vi "PI Terminal.vi"() -> ()   [LabVIEW 2014]
doc: "HELP for Terminal.vi\n\nThe terminal VI is a stand-alone application. It first asks the user to specify the full configuration (number of controlled systems, RS-232, GPIB, TCP-IP or DLL communication, communications parameters), then it establishes a connection with a selected system. This will work for all PI devices which support the PI General Command Set, or at least follow the same syntax rules and support the *IDN? and ERR? commands.\n\nAfter starting the VI, the interface parameters of the systems with which to communicate must be selected. For this reason, \"PITerminal.vi\" calls \"PI Ask for Communication Parameters.vi\". Select here the number of connected PI systems that you want to communicate with. For each system, select the appropriate interface parameters. \n\nC-413: Interface = RS232, DLL, or TCP/IP. TCP/IP support available depending on controller version! If unsure whether your controller supports TCP/IP communication, please refer to the controller user manual), RS232: Input and output HW handshake must be TRUE. DLL: DLL for Device = PI_GCS2_DLL, DLL Interface = USB, Parameter = Serial no. of system to connect to. Syntax: GCS 2.0; Term char = LF.\n\nC-702: Interface = RS232 or TCP/IP, RS232: Input and output HW handshake must be TRUE. Syntax: GCS 1.0; Term char = LF.\n\nC-843: Interface = DLL, DLL for Device = C-843, DLL Interface = Board, Parameter = Board number (1 for first C-843 board). Syntax: GCS 1.0; Term char = LF.\n\nC-843.PM: Interface = DLL, DLL for Device = C-843.PM, DLL Interface = Board, Parameter = Board number (1 for first C-843 board). Syntax: GCS 1.0; Term char = LF.\n\nC-844: Interface = DLL, DLL for Device = C-844, DLL Interface = RS232 or GPIB, Parameter = empty string, RS232 baud rate = 9600. Syntax: GCS 1.0; Term char = LF.\n\nC-865: Interface = DLL, DLL for Device = C-865, DLL Interface = RS232, Parameter = empty string, RS232 baud rate = set as appropriate. Syntax: GCS 1.0; Term char = LF.\n\nC-866: Interface = DLL, DLL for Device = C-866, DLL Interface = RS232 or USB, RS232: Parameter = empty string, RS232 baud rate = set as appropriate, USB: Parameter = Serial no. of system to connect to, Syntax: GCS 1.0; Term char = LF.\n\nC-867: Single Device: Interface = RS232, TCP/IP or DLL, RS232: Input and output HW handshake must be FALSE. DLL (USB): DLL for Device = C-867, DLL Interface = USB, Parameter = Serial no. of system to connect to. DaisyChain: Interface = DLL, DLL for Device = C-867, DLL Interface = RS232_DC, Parameter = Number of device in chain, Register DC: FALSE. Syntax: GCS 2.0; Term char = LF.\n\nC-877: Interface = RS232 or DLL, RS232: Input and output HW handshake must be FALSE. DLL (USB): DLL for Device = PI_GCS2_DLL, DLL Interface = USB, Parameter = Serial no. of system to connect to. Syntax: GCS 2.0; Term char = LF.\n\nC-880, C-848: Interface = RS232 or GPIB, RS232: Input and output HW handshake must be TRUE. Syntax: GCS 1.0; Term char = LF.\n\nC-880K005: Interface = RS232, Input and output HW handshake must be FALSE. Syntax: GCS 1.0; Term char = LF.\n\nC-884: Interface = RS232, TCP/IP or DLL, RS232: Input and output HW handshake must be FALSE. DLL (USB): DLL for Device = PI_GCS2_DLL, DLL Interface = USB, Parameter = Serial no. of system to connect to. Syntax: GCS 2.0; Term char = LF.\n\nC-885: Interface = TCP/IP or DLL. DLL (USB): DLL for Device = PI_GCS2_DLL, DLL Interface = USB, Parameter = Serial no. of system to connect to. Syntax: GCS 2.0; Term char = LF.DaisyChain: Interface = DLL, DLL for Device = PI_GCS2_DLL, DLL Interface = TCPIP_DC or USB_DC, Parameter = Number of device in chain, Register DC: FALSE. Syntax: GCS 2.0; Term char = LF.\n\nC-886: Interface = TCP/IP or DLL. DLL (USB): DLL for Device = PI_GCS2_DLL, DLL Interface = USB, Parameter = Serial no. of system to connect to. Syntax: GCS 2.0; Term char = LF.\n\nC-887, F-206, M-8X0: For GCS syntax version = GCS 1.0 (older firmware or compatibility mode, can be set with CSV.vi), Interface = RS232, GPIB (not available for C-887 controller) or TCP/IP., The error status will not be cleared by this VI. The first ERR? query will report a hidden error with error code 1, which will be cleared during system initialization (INI). RS232: Input and output handshake settings must be FALSE. Syntax: GCS 1.0; Term char = LF.\nFor GCS syntax version = GCS 2.0 (C-887 Controller), Interface = RS232 or TCP/IP. RS232: Input and output handshake settings must be FALSE. Syntax: GCS 2.0; Term char = LF.\n\nC-891: Interface = RS232, TCP/IP or DLL. TCP/IP support available depending on controller version! If unsure whether your controller supports TCP/IP communication, please refer to your user manual. RS232: Input and output HW handshake must be FALSE. DLL (USB): DLL for Device = PI_GCS2_DLL, DLL Interface = USB, Parameter = Serial no. of system to connect to. Syntax: GCS 2.0; Term char = LF.\n\nE-516: Interface = RS232 or GPIB, RS232: Input and output HW handshake must be TRUE. Syntax: GCS 1.0; Term char = LF.\n\nE-517: Interface = RS232, GPIB, TCP/IP or DLL, RS232: Input and output HW handshake must be TRUE, DLL (USB): DLL for Device = E-517, DLL Interface = USB, Parameter = Serial no. of system to connect to. Syntax: GCS 2.0; Term char = LF.\n\nE-518: Interface = RS232, TCP/IP or DLL, RS232: Input and output HW handshake must be TRUE, DLL (USB): DLL for Device = PI_GCS2_DLL, DLL Interface = USB, Parameter = Serial no. of system to connect to. Syntax: GCS 2.0; Term char = LF.\n\nE-709: Interface = RS232 or DLL, RS232: Input and output HW handshake must be TRUE. DLL (USB): DLL for Device = E-709, DLL Interface = USB, Parameter = Serial no. of system to connect to. Syntax: GCS 2.0; Term char = LF.\n\nE-710: Interface = DLL, DLL for Device = E-710, DLL Interface = RS232 or GPIB, Parameter = empty string. Syntax: GCS 1.0; Term char = LF.\n\nE-712: Interface = RS232, TCP/IP or DLL, RS232: Input and output HW handshake must be TRUE. DLL: DLL for Device = E-712, DLL Interface = USB, Parameter = Serial no. of system to connect to. Syntax: GCS 2.0; Term char = LF.\n\nE-725: Interface = RS232, TCP/IP or DLL, RS232: Input and output HW handshake must be TRUE. DLL: DLL for Device = E-725, DLL Interface = USB, Parameter = Serial no. of system to connect to. Syntax: GCS 2.0; Term char = LF.\n\nE-727: Interface = RS232, TCP/IP or DLL, RS232: Input and output HW handshake must be TRUE. DLL: DLL for Device = PI_GCS2_DLL, DLL Interface = USB,Parameter = Serial no. of system to connect to. Syntax: GCS 2.0; Term char = LF.\n\nE-753: Interface = RS232 or TCP/IP, RS232: Input and output HW handshake must be TRUE. Syntax: GCS 2.0; Term char = LF.\n\nE-754: Interface = RS232, TCP/IP or DLL, RS232: Input and output HW handshake must be TRUE. DLL: DLL for Device = E-754, DLL Interface = USB, Parameter = Serial no. of system to connect to. Syntax: GCS 2.0; Term char = LF.\n\nE-755: Single Device: Interface = RS232, Input and output HW handshake must be TRUE. DaisyChain: Interface = DLL, DLL for Device = E-755, DLL Interface = RS232_DC, Parameter = Number of device in chain (first device: 1). Syntax: GCS 2.0; Term char = LF.\n\nE-761: Interface = DLL, DLL for Device = E-761, DLL Interface = Board, Parameter = Board number (1 for first E-761 board). Syntax: GCS 1.0; Term char = LF.\n\nE-816: Interface = RS232 or DLL, RS232: Input and output HW handshake must be TRUE. DLL (USB): DLL for Device = E-816, DLL Interface = USB, Parameter = Serial no. of system to connect to. Syntax: GCS 1.0; Term char = LF. \n\nE-861: Single Device: Interface = RS232 or DLL, RS232: Input and output HW handshake must be FALSE. DLL (USB): DLL for Device = E-861, DLL Interface = USB, Parameter = Serial no. of system to connect to. DaisyChain: Interface = DLL, DLL for Device = E-861, DLL Interface = RS232_DC, Parameter = Number of device in chain (first device: 1), Register DC: FALSE. Syntax: GCS 2.0; Term char = LF.\n\nE-870: Interface = DLL, DLL (USB): DLL for Device = PI_GCS2_DLL, DLL Interface = USB, Parameter = Serial no. of system to connect to.\nSyntax: GCS 2.0; Term char = LF.\n\nE-871: Single Device: Interface = RS232 or DLL, RS232: Input and output HW handshake must be FALSE. DLL (USB): DLL for Device = PI_GCS2_DLL, DLL Interface = USB, Parameter = Serial no. of system to connect to.\nDaisyChain: Interface = DLL, DLL for Device = PI_GCS2_DLL, DLL Interface = RS232_DC or USB_DC, Parameter = Number of device in chain, Register DC: FALSE. Syntax: GCS 2.0; Term char = LF.\n\nE-872: Interface = RS232, TCP/IP or DLL, RS232: Input and output HW handshake must be FALSE. DLL (USB): DLL for Device = PI_GCS2_DLL, DLL Interface = USB, Parameter = Serial no. of system to connect to. Syntax: GCS 2.0; Term char = LF.\n\nE-873: Interface = RS232, TCP/IP or DLL, RS232: Input and output HW handshake must be FALSE. DLL (USB): DLL for Device = PI_GCS2_DLL, DLL Interface = USB, Parameter = Serial no. of system to connect to. Syntax: GCS 2.0; Term char = LF.\n\nE-874: Interface = RS232, TCP/IP or DLL, RS232: Input and output HW handshake must be FALSE. DLL (USB): DLL for Device = PI_GCS2_DLL, DLL Interface = USB, Parameter = Serial no. of system to connect to. Syntax: GCS 2.0; Term char = LF.\n\nHydra: Interface = DLL, DLL (TCP/IP and RS-232): DLL for Device = PI_HydraPollux_GCS2_DLL, DLL Interface = RS232 or TCP/IP, Syntax: GCS 2.0; Term char = LF.\n\nMercury™: Interface = DLL, DLL for Device = Mercury™, DLL Interface = RS232 (even if using USB), Parameter = empty string, RS232 baud rate = same as set on controller hardware. Syntax: GCS 1.0; Term char = LF.\n\nGCS_Mercury: Single Device: Interface = RS232 or DLL, RS232: Input and output HW handshake must be FALSE. DLL (USB): DLL for Device = PI_GCS2_DLL, DLL Interface = USB, Parameter = Serial no. of system to connect to.\nDaisyChain: Interface = DLL, DLL for Device = PI_GCS2_DLL, DLL Interface = RS232_DC, Parameter = Number of device in chain, Register DC: FALSE. Syntax: GCS 2.0; Term char = LF.\n\nPollux: Interface = DLL, DLL (RS-232): DLL for Device = PI_HydraPollux_GCS2_DLL, DLL Interface = RS232, Baudrate must be 19200, Syntax: GCS 2.0; Term char = LF.\n\nIf the chosen timeout value is greater than 1000 ms, it will automatically be set to 1000 ms for a fluid program operation. \n\nIn the upper window (\"Send\") the user can enter commands which will be transmitted to the chosen device one line at a time when the ENTER key is pressed. \nAll controller responses are displayed in the Receive response window, which can be cleared by pressing the Clear Receive Window button or F2. \n\nThe view style of the Receive window can be changed to Show all characters or Hex View using the menu ring above the Receive window.\n\nExit or F10 will terminate the terminal application. \n\nTo send the last command again, just press the ENTER key again. The next line will then show the following entry: \"(Send: cmd)\" with cmd being the command from the line before, which was resent.\n\nWhen the terminal application has just been started, pressing ENTER without entering a command will send \"*IDN?\" to the chosen system. \n\nNew commands can only be inserted into the last line of the Send window. The user can scroll through the history of the Send window using the scroll bar or the cursor up/down keys, but cannot change the history or resend commands by pressing ENTER unless in the last line. Pressing ENTER will always resend the last command, no matter where the cursor is positioned. Selecting text and using copy and paste (Ctrl+C, Ctrl+V) works for single lines, if only the contents of one single line (the command text) is selected and copied, not the full line (including the LineFeed) or multiple lines.\n\nMany of PI's General Command Set compatible devices support single-byte commands. For example, the user can stop a fast scan of a C-880 or C-887by sending an ASCII 24 (decimal). To enter this command into the Send window simply type a \"#\" followed by the decimal value of the byte to be sent, e.g. enter \"#24\" and presses ENTER to stop a fast scan. An entry \"(Send: *)\" will be added to the original command with * being the corresponding ASCII character of the single byte sent. \n\nPressing F1 or the Help button will pop up a help window. To return to the terminal application, press Esc. If Send ERR? on Exit? is TRUE, an \"ERR?\" query is sent to the device when Exit is pressed to prevent the controller from keeping an error condition produced during the use of the terminal application."
uses:
  Low Level/Communication.llb/Termination character.ctl
  Low Level/Communication.llb/Available DLLs.ctl
  Low Level/Communication.llb/Global DaisyChain.vi
panel:
  out "Help string":string="\nHELP for PI Terminal.vi\nPress Esc to return to the terminal application.\n\nThis terminal application works for all PI devices which support the PI General Command Set or at least follow the syntax rules of this command structure and support the commands *IDN? and ERR?.\n\nIn the upper window (\"Send\") the user can enter commands which will be transmitted to the chosen device one line at a time when the ENTER key is pressed. All controller responses are displayed in the Receive response window, which can be cleared by pressing the Clear Receive Window button or F2. The view style of the Receive window can be changed to Show all characters or Hex View using the menu ring above the Receive window.\n\nExit or F10 will terminate the terminal application. \n\nTo send the last command again, just press the ENTER key again. The next line will then show the following entry: \"(Send: cmd)\" with cmd being the command from the line before, which was resent.\nWhen the terminal application has just been started, pressing ENTER without entering a command will send \"*IDN?\" to the chosen system.\n\nNew commands can only be inserted into the last line of the Send window. The user can scroll through the history of the Send window using the scroll bar or the cursor up/down keys, but cannot change the history or resend commands by pressing ENTER unless in the last line. Pressing ENTER will always resend the last command, no matter where the cursor is positioned. Selecting text and using copy and paste (Ctrl+C, Ctrl+V) works for single lines, if only the contents of one single line (the command text) is selected and copied, not the full line (including the LineFeed) or multiple lines.\n\nMany of PI's General Command Set compatible devices support single-byte commands. For example, the user can stop a fast scan of a C-880 or F-206 by sending an ASCII 24 (decimal). To enter this command into the Send window simply type a \"#\" followed by the decimal value of the byte to be sent, e.g. enter \"#24\" and presses ENTER to stop a fast scan. An entry \"(Send: *)\" will be added to the original command with * being the corresponding ASCII character of the single byte sent. \n\nIf Send ERR? on Exit? is TRUE, a \"ERR?\" query is sent to the device when Exit is pressed to prevent the controller from keeping an error condition produced during the use of the terminal application.\n\nC-413: \tInterface = RS232, DLL, or TCP/IP. TCP/IP support available depending on controller version! If unsure whether your controller supports TCP/IP communication, please refer to the controller user manual), RS232: Input and output HW handshake must be TRUE. DLL: DLL for Device = PI_GCS2_DLL, DLL Interface = USB, Parameter = Serial no. of system to connect to. Syntax: GCS 2.0; Term char = LF.\n\nC-414: \tInterface = RS232, DLL, or TCP/IP. RS232: Input and output HW handshake must be TRUE. DLL: DLL for Device = PI_GCS2_DLL, DLL Interface = USB, Parameter = Serial no. of system to connect to. Syntax: GCS 2.0; Term char = LF.\n\nC-702: \tInterface = RS232 or TCP/IP, RS232: Input and output HW handshake \tmust \tbe TRUE. Syntax: GCS 1.0; Term char = LF.\n\nC-843: \tInterface = DLL, DLL for Device = C-843, DLL Interface = Board, \tParameter = Board number (1 for first C-843 board). Syntax: GCS 1.0; \tTerm char = LF.\n\nC-843.PM: \tInterface = DLL, DLL for Device = C-843.PM, DLL Interface = Board, \tParameter = Board number (1 for first C-843 board). Syntax: GCS 1.0; \tTerm char = LF.\n\nC-865: \tInterface = DLL, DLL for Device = C-865, DLL Interface = RS232, \tParameter = empty string, RS232 baud rate = set as appropriate. Syntax: \tGCS 1.0; Term char = LF.\n\nC-866: \tInterface = DLL, DLL for Device = C-866, DLL Interface = RS232 or USB, \tRS232: Parameter = empty string, RS232 baud rate = set as appropriate, \tUSB: Parameter = Serial no. of system to connect to, \n\tSyntax: GCS 1.0; Term char = LF.\n\nC-867: \tSingle Device: Interface = RS232, TCP/IP or DLL, RS232: Input and output HW \thandshake must be FALSE. DLL (USB): DLL for Device = C-867, DLL \tInterface = USB, Parameter = Serial no. of system to connect to.\nDaisyChain: Interface = DLL, DLL for Device = C-867, DLL Interface = \tRS232_DC, Parameter = Number of device in chain, \tRegister DC: \tFALSE. Syntax: GCS 2.0; Term char = LF.\n\nC-880, C-848: \tInterface = RS232 or GPIB, RS232: Input and output HW handshake must \tbe TRUE. Syntax: GCS 1.0; Term char = LF.\n\nC-880K005: \tInterface = RS232, Input and output HW handshake must be FALSE. \tSyntax: GCS 1.0; Term char = LF.\n\nC-884: \tInterface = RS232, TCP/IP or DLL, RS232: Input and output HW handshake must be FALSE. DLL (USB): DLL for Device = PI_GCS2_DLL, DLL Interface = USB, Parameter = Serial no. of system to connect to. Syntax: GCS 2.0; Term char = LF.\n\nC-885: \tInterface = TCP/IP or DLL. DLL (USB): DLL for Device = PI_GCS2_DLL, DLL Interface = USB, Parameter = Serial no. of system to connect to. Syntax: GCS 2.0; Term char = LF.\nDaisyChain: Interface = DLL, DLL for Device = PI_GCS2_DLL, DLL Interface = \tTCPIP_DC or USB_DC, Parameter = Number of device in chain, \tRegister DC: \tFALSE. Syntax: GCS 2.0; Term char = LF.\n\nC-886: \tInterface = TCP/IP or DLL. DLL (USB): DLL for Device = PI_GCS2_DLL, DLL Interface = USB, Parameter = Serial no. of system to connect to. Syntax: GCS 2.0; Term char = LF.\n\nC-887, F-206, M-8X0: \tFor GCS syntax version = GCS 1.0 (older firmware or compatibility mode, \tcan be set with CSV.vi), Interface = RS232, GPIB (not available for C-887 \tcontroller) or TCP/IP., The error status will not be cleared by this VI. The \tfirst ERR? query will report a hidden error with error code 1, which will be \tcleared during system initialization (INI). RS232: Input and output \thandshake settings must be FALSE. Syntax: GCS 1.0; Term char = \tLF.\n\tFor GCS syntax version = GCS 2.0 (C-887 Controller), Interface = RS232 \tor TCP/IP. RS232: Input and output handshake settings must be FALSE. \tSyntax: GCS 2.0; Term char = LF.\n\nC-891: \tInterface = RS232, TCP/IP or DLL. TCP/IP support available depending on \tcontroller version! If unsure whether your controller supports TCP/IP \tcommunication, please refer to your user manual. RS232: Input and output \tHW handshake must be FALSE. DLL (USB): DLL for Device = \tPI_GCS2_DLL, DLL Interface = USB, Parameter = Serial no. of system to \tconnect to. Syntax: GCS 2.0; Term char = LF.\n\nE-516: \tInterface = RS232 or GPIB, RS232: Input and output HW handshake must \tbe TRUE. Syntax: GCS 1.0; Term char = LF.\n\nE-517: \tInterface = RS232, GPIB, TCP/IP or DLL, RS232: Input and output HW \thandshake must be TRUE, DLL (USB): DLL for Device = E-517, DLL \tInterface = USB, Parameter = Serial no. of system to connect to. \nSyntax: GCS 2.0; Term char = LF.\n\nE-518: \t\tInterface = RS232, TCP/IP or DLL, RS232: Input and output HW handshake must be TRUE, DLL (USB): DLL for Device = PI_GCS2_DLL, DLL Interface = USB, Parameter = Serial no. of system to connect to. \nSyntax: GCS 2.0; Term char = LF.\n\nE-709: \tInterface = RS232 or DLL, RS232: Input and output HW handshake \tmust be TRUE. DLL (USB): DLL for Device = E-709, DLL Interface = USB, \tParameter = Serial no. of system to connect to. Syntax: GCS 2.0; Term \tchar = LF.\n\nE-710:\tInterface = DLL, DLL for Device = E-710, DLL Interface = RS232 or GPIB, \tParameter = empty string. Syntax: GCS 1.0; Term char = LF.\n\nE-712: \tInterface = RS232, TCP/IP or DLL, RS232: Input and output HW \thandshake must be TRUE. DLL: DLL for Device = E-712, DLL Interface = \tUSB, \tParameter = Serial no. of system to connect to. \n\tSyntax: GCS 2.0; Term char = LF.\n\nE-725: \tInterface = RS232, TCP/IP or DLL, RS232: Input and output HW \thandshake must be TRUE. DLL: DLL for Device = E-725, DLL Interface = \tUSB, \tParameter = Serial no. of system to connect to. \nSyntax: GCS 2.0; Term char = LF.\n\nE-727: \tInterface = RS232, TCP/IP or DLL, RS232: Input and output HW \thandshake must be TRUE. DLL: DLL for Device = PI_GCS2_DLL, DLL Interface = \tUSB, \tParameter = Serial no. of system to connect to. \tSyntax: GCS 2.0; Term char = LF.\n\nE-753: \tInterface = RS232 or TCP/IP, RS232: Input and output HW handshake \tmust \tbe TRUE. Syntax: GCS 2.0; Term char = LF.\n\nE-754: Interface = RS232, TCP/IP or DLL, RS232: Input and output HW handshake must be TRUE. DLL: DLL for Device = E-754, DLL Interface = USB, Parameter = Serial no. of system to connect to. Syntax: GCS 2.0; Term char = LF.\n\nE-755:\tSingle Device: Interface = RS232, Input and output HW handshake must \tbe TRUE. DaisyChain: Interface = DLL, DLL for Device = E-755, DLL \tInterface = RS232_DC, Parameter = Number of device in chain (first \tdevice: 1). Syntax: GCS 2.0; Term char = LF.\n\nE-761:\tInterface = DLL, DLL for Device = E-761, DLL Interface = Board, \tParameter = Board number (1 for first E-761 board). Syntax: GCS 1.0; \tTerm char = LF.\n\nE-816: \tInterface = RS232 or DLL, RS232: Input and output HW handshake must \tbe TRUE. DLL (USB): DLL for Device = E-816, DLL Interface = USB, \tParameter = Serial no. of system to connect to. Syntax: GCS 1.0; Term \tchar = LF. \n\nE-861: \tSingle Device: Interface = RS232 or DLL, RS232: Input and output HW \thandshake must be FALSE. DLL (USB): DLL for Device = E-861, DLL \tInterface = USB, Parameter = Serial no. of system to connect to.\nDaisyChain: Interface = DLL, DLL for Device = E-861, DLL Interface = \tRS232_DC or USB_DC, Parameter = Number of device in chain (first device: 1), \tRegister DC: FALSE. Syntax: GCS 2.0; Term char = LF.\n\nE-870: \tInterface = DLL, DLL (USB): DLL for Device = PI_GCS2_DLL, DLL \tInterface = USB, Parameter = Serial no. of system to connect to.\n\tSyntax: GCS 2.0; Term char = LF.\n\nE-871: Single Device: Interface = RS232 or DLL, RS232: Input and output HW \thandshake must be FALSE. DLL (USB): DLL for Device = \tPI_GCS2_DLL, DLL Interface = USB, Parameter = Serial no. of system to \tconnect to.\n\tDaisyChain: Interface = DLL, DLL for Device = PI_GCS2_DLL, DLL \tInterface = RS232_DC or USB_DC, Parameter = Number of device in \tchain, Register DC: FALSE. Syntax: GCS 2.0; Term char = LF.\n\nE-872: Interface = RS232, TCP/IP or DLL: Input and output HW \thandshake must be FALSE. DLL (USB): DLL for Device = \tPI_GCS2_DLL, DLL Interface = USB, Parameter = Serial no. of system to \tconnect to. Syntax: GCS 2.0; Term char = LF.\n\nE-873: Interface = RS232, TCP/IP or DLL, RS232: Input and output HW handshake must be FALSE. DLL (USB): DLL for Device = PI_GCS2_DLL, DLL Interface = USB, Parameter = Serial no. of system to \tconnect to. Syntax: GCS 2.0; Term char = LF.\n\nE-874: Interface = RS232, TCP/IP or DLL, RS232: Input and output HW handshake must be FALSE. DLL (USB): DLL for Device = PI_GCS2_DLL, DLL Interface = USB, Parameter = Serial no. of system to \tconnect to. Syntax: GCS 2.0; Term char = LF.\n\nHydra: \tInterface = DLL, DLL (TCP/IP and RS-232): DLL for Device = \t\t\t\t\tPI_HydraPollux_GCS2_DLL, DLL Interface = RS232 or TCP/IP, Syntax: \t\t\tGCS 2.0; Term char = LF.\n\nMercury™: \tInterface = DLL, DLL for Device = Mercury™, DLL Interface = RS232 \t(even if using USB), Parameter = empty string, RS232 baud rate = same \tas set on controller hardware, Syntax: GCS 1.0; Term char = LF.\n\nGCS_Mercury: \tSingle Device: Interface = RS232 or DLL, RS232: Input and output HW \thandshake must be FALSE. DLL (USB): DLL for Device = PI_GCS2_DLL, \tDLL Interface = USB, Parameter = Serial no. of system to connect to. \tDaisyChain: Interface = DLL, DLL for Device = PI_GCS2_DLL, DLL \tInterface = RS232_DC or USB_DaisyChain, Parameter = Number of device in chain, \tRegister DC: \tFALSE. Syntax: GCS 2.0; Term char = LF.\n\nPollux: \tInterface = DLL, DLL (RS-232): DLL for Device = PI_HydraPollux_GCS2_DLL, \t\tDLL Interface = RS232, Baudrate must be 19200, Syntax: GCS 2.0; Term char = LF.\n\n"
  in  "HowTo":string="Start application and choose interface parameters in next window."
  out "TCP/IP Config. System":T1={"Host address/name"="Z-A521-2.pi.ws", "Port"=3000, "Board"=0, "Timeout"=5000}
  in  "ERR? on exit?":bool=TRUE
  out "error out":T2
  out "GPIB Configuration system":T3={"bus"=0, "address"=4, "mode"=0, "Timeout"=1000}
  in  "Hide help":bool
  in  "Show help":bool
  in  "View style":u16(ring) items=["Normal view", "Show all characters", "Hex View"]
  out "error":bool
  in  "Send":bool
  in  "Clear":bool
  in  "Exit":bool
  out "Receive":string
  in  "System No.":i32=1 min=1 step=1
  out "Interface":u16(ring) items=["RS232", "GPIB", "DLL", "TCP/IP"]
  out "System ind.":i32=1
  out "System":i32=1
  out "RS232 Config. System":T4={"RS232 Portnumber"=0, "Timeout"=1000, "Baudrate"=57600, "Handshake"=0} {"Handshake" items=["None", "HW", "XON/XOFF"]; "RS232 Portnumber" items=["COM1", "COM2", "COM3", "COM4", "COM5", "COM6", "COM7", "COM8", "COM9", "COM10", "COM11", "COM12", "COM13", "COM14", "COM15", "COM16", "COM17", "COM18", "COM19", "COM20", "COM21", "COM22", "COM23", "COM24", "COM25", "COM26", "COM27", "COM28", "COM29", "COM30"]}
  in  "Send":string="*IDN?\n"
  out "Term.char":T5
  out "DLL for Device":T6=17 items=["C-843", "C-844", "E-710", "C-843.PM", "C-865", "E-761", "Mercury", "E-755", "E-753", "C-866", "E-712", "E-725", "E-861", "C-867", "E-517", "E-816", "E-709", "PI_GCS2_DLL", "HydraPollux"]
  # "Terminal"
  # "If chosen timeout value is > 1000 ms, \nit will be set to 300 ms."
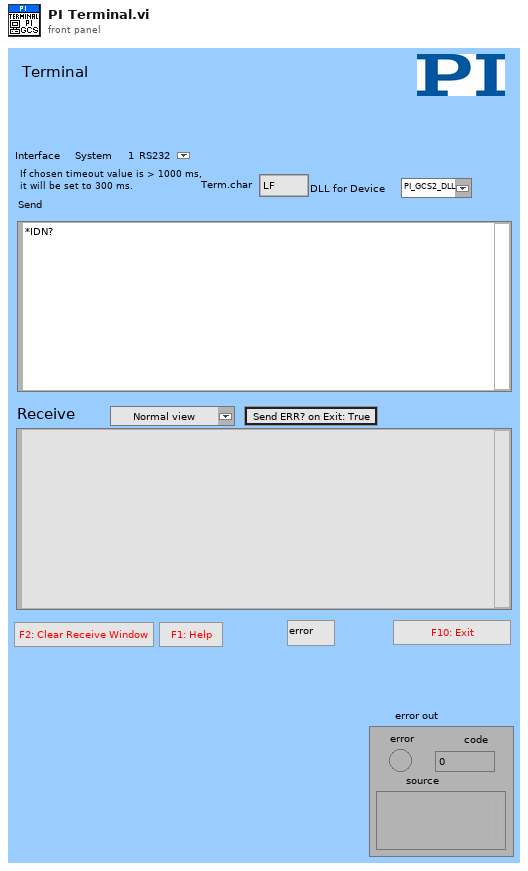
[diagram p1: front panel]
types:
  T1 = cluster{"Host address/name":string, "Port":i32, "Board":i32, "Timeout":i32}
  T2 = cluster{"error":bool, "code":i32, "source":string}
  T3 = cluster{"bus":i16, "address":i16, "mode":i16, "Timeout":i32}
  T4 = cluster{"RS232 Portnumber":i32, "Timeout":i32, "Baudrate":u32, "Handshake":u16}
  T5 = typedef "Termination character.ctl" = enum16{"LF", "CR", "LFCR", "CRLF"}
  T6 = typedef "Available DLLs.ctl" = u16
  T7 = cluster{"data bits":u16, "stop bits":enum16{"1 bit", "1.5 bits", "2 bits"}, "parity":enum16{"no parity", "odd parity", "even parity", "mark parity", "space parity"}}
  T8 = cluster{"Host address/name":string, "Port":i32, "Board":i32}[]
  T9 = cluster{"input XON/XOFF":bool, "input HW Handshake":bool, "input alt HW HShk":bool, "output XON/XOFF":bool, "output HW Handshake":bool, "output alt HW HShk":bool, "XOFF byte ":u8, "XON byte":u8, "parity error byte":u16}[]
  T10 = typedef "Available interfaces.ctl" = u16
  T11 = cluster{"RS232 Portnumber":u16, "Timeout":u32, "RS232 baud rate":u32, "Interface":T10, "GPIB Bus":i16, "GPIB address":i16, "GPIB Mode":i16}[]
  T12 = typedef "Available DLL interfaces.ctl" = u16
  T13 = cluster{"DLL for Device":T6, "DLL Interface":T12, "Parameter":string}[]
  T14 = cluster{"No. of devices":i32, "Port ID":i32, "Devices":string[], "Description":string}[]
  T15 = cluster{"No. of devices":i32, "Port ID":i32, "Devices":string[], "Description":string}
  T16 = cluster{"DLL for Device":T6, "DLL Interface":T12, "Parameter":string}
  T17 = cluster{"RS232 Portnumber":u16, "Timeout":u32, "RS232 baud rate":u32, "Interface":T10, "GPIB Bus":i16, "GPIB address":i16, "GPIB Mode":i16}
  T18 = cluster{"Portnumber":u32, "Timeout":i32, "Baudrate":u32, "Handshake":u16}
  T19 = cluster{"data bits":u16, "stop bits":enum16{"1 bit", "1.5 bits", "2 bits"}, "parity":enum16{"no parity", "odd parity", "even parity", "mark parity", "space parity"}}[]
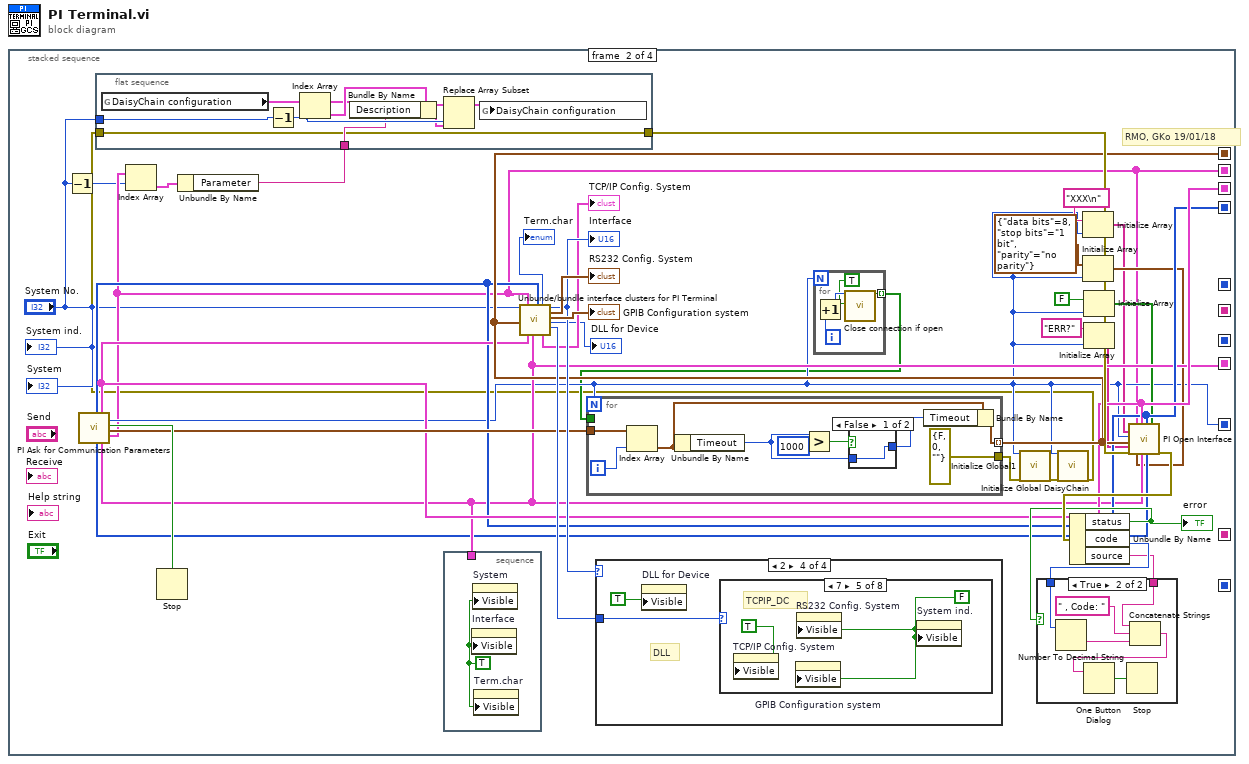
[diagram p0: block diagram]
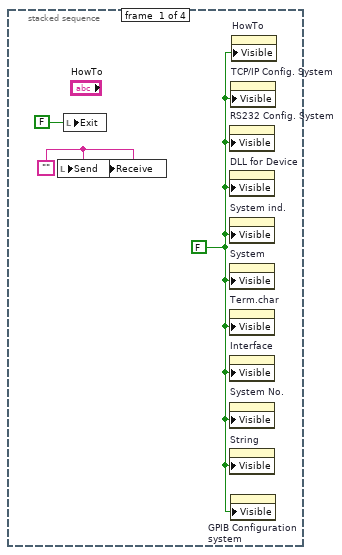
[diagram p2: hidden frame]
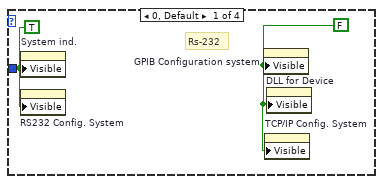
[diagram p3: hidden frame]
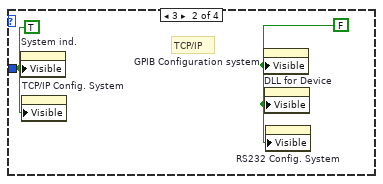
[diagram p4: hidden frame]
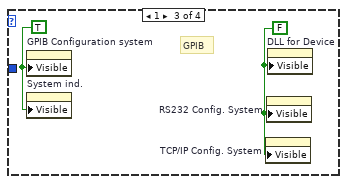
[diagram p5: hidden frame]
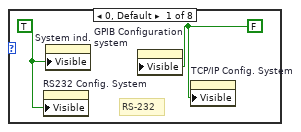
[diagram p6: hidden frame]
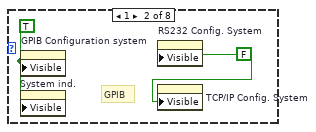
[diagram p7: hidden frame]
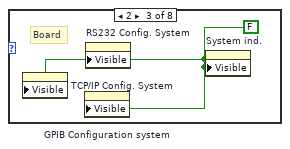
[diagram p8: hidden frame]
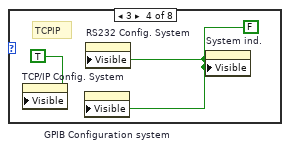
[diagram p9: hidden frame]
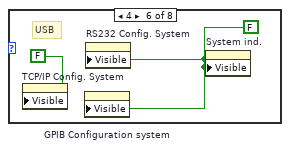
[diagram p10: hidden frame]
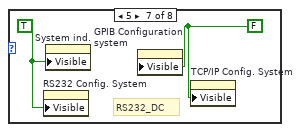
[diagram p11: hidden frame]
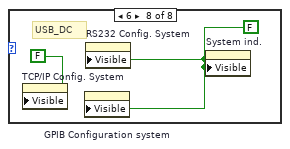
[diagram p12: hidden frame]
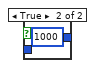
[diagram p14: hidden frame]
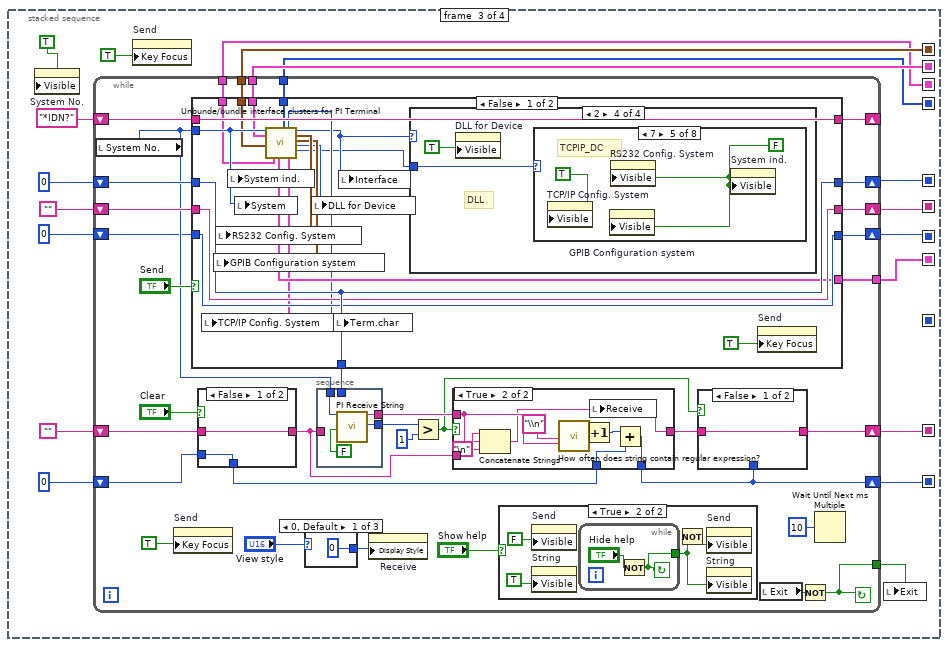
[diagram p15: hidden frame]
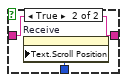
[diagram p17: hidden frame]
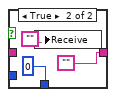
[diagram p18: hidden frame]
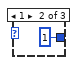
[diagram p20: hidden frame]
diagram:
  n1 = stacked-sequence {
    seq-local: [_ w29 _ _] -> [_ _ w111 _]
    seq-local: [_ w9 _ _] -> [_ _ w110 _]
    seq-local: [_ w24 _ _] -> [_ _ w101 _]
    seq-local: [_ _ w100 _] -> [_ _ _ w262]
    seq-local: [_ _ w99 _] -> [_ _ _ w261]
    seq-local: [_ _ w98 _] -> [_ _ _ w263]
    seq-local: [_ _ w97 _] -> [_ _ _ w264]
    seq-local: [_ _ w96 _] -> [_ _ _ w265]
    seq-local: [_ w26 _ _] -> [_ _ w95 _]
    seq-local: [_ w25 _ _] -> [_ _ w94 _]
    seq-local: [_ w13 _ _] -> [_ _ _ w259]
    frame #0 {
      w1 = FALSE ("Visible")
      w3 = ""
      n2 = local write "Send"(w3) -> ()
      n3 = local write "Exit"(FALSE ("error")) -> ()
      n4 = local write "Receive"(w3) -> ()
      n5 = property on="RS232 Config. System" class="Clust (strict)"("Visible"=w1) -> ()  [unwired: 2 in, 2 out]
      n6 = property on="DLL for Device" class="Ring (strict)"("Visible"=w1) -> ()  [unwired: 2 in, 2 out]
      n7 = property on="System ind." class="DigNum (strict)"("Visible"=w1) -> ()  [unwired: 2 in, 2 out]
      n8 = property on="System" class="DigNum (strict)"("Visible"=w1) -> ()  [unwired: 2 in, 2 out]
      n9 = property on="Term.char" class="Enum (strict)"("Visible"=w1) -> ()  [unwired: 2 in, 2 out]
      n10 = property on="Interface" class="Ring (strict)"("Visible"=w1) -> ()  [unwired: 2 in, 2 out]
      n11 = property on="System No." class="DigNum (strict)"("Visible"=w1) -> ()  [unwired: 2 in, 2 out]
      n12 = property on="String" class="Str"("Visible"=w1) -> ()  [unwired: 2 in, 2 out]
      n13 = property on="TCP/IP Config. System" class="Clust (strict)"("Visible"=w1) -> ()  [unwired: 2 in, 2 out]
      n14 = property on="GPIB Configuration system" class="Clust (strict)"("Visible"=w1) -> ()  [unwired: 2 in, 2 out]
      n15 = property on="HowTo" class="Str"("Visible"=w1) -> ()  [unwired: 2 in, 2 out]
    }
    frame #1 {
      # "RMO, GKo 19/01/18"
      n16 = Decrement(x="System No.") -> (x-1=w8:i32)
      n17 = call "PI Ask for Communication Parameters.vi"() -> ("Termination character out"=w25:T5[], "Syntax out"=w23:enum16{"GCS 1.0", "GCS 2.0"}[], "TCP/IP Configuration out"=w26:T8, "Flow control out"=w24:T9, "How many\nsystems? out"=w13:i32, "Abort out"=w38:bool, "Interface configuration out"=w30:T11, "DLL Interface\nconfiguration out"=w9:T13)  [unwired: 12 out]
      n18 = flat-sequence {
        tunnel: "System No." -> [w43]
        tunnel: w5 -> [w42]
        tunnel: w4 -> [w41]
        tunnel: [w41] -> w40
        frame #0 {
          n19 = global read "Global DaisyChain.vi" "DaisyChain configuration"() -> (w47:T14)
          n20 = Decrement(x=w43) -> (x-1=w46:i32)
          n21 = Index Array(array=w47, index=w46) -> (element=w48:T15)
          n22 = Bundle By Name(cluster=w48, "Description"=w42) -> (w45:T15)
          n23 = Replace Array Subset(array=w47, new element=w45, index=w46) -> (w44:T14)
          n24 = global write "Global DaisyChain.vi" "DaisyChain configuration"(w44) -> ()
        }
      }
      n25 = Index Array(array=w9, index=w8) -> (element=w6:T16)
      n26 = Stop(stop? (T)=w38) -> ()
      n27 = Unbundle By Name(w6) -> ("Parameter"=w5:string)
      n28 = stacked-sequence {
        tunnel: w24 -> [_]
        frame #0 {
          w53 = TRUE ("Visible")
          n29 = property on="Interface" class="Ring (strict)"("Visible"=w53) -> ()  [unwired: 2 in, 2 out]
          n30 = property on="System" class="DigNum (strict)"("Visible"=w53) -> ()  [unwired: 2 in, 2 out]
          n31 = property on="Term.char" class="Enum (strict)"("Visible"=w53) -> ()  [unwired: 2 in, 2 out]
        }
      }
      n32 = for {
        N: w13 -> [_]
        tunnel: [w49] -> w12 mode=indexing
        i -> [w52]
        n33 = Increment(x=w52) -> (x+1=w51:i32)
        n34 = call "Close connection if open.vi"("System no."=w51, "Close DaisyChain"=TRUE) -> ("Was connected?"=w49:bool)  [unwired: 1 in, 16 out]
      }
      n35 = for {
        N: w13 -> [_]
        tunnel: w30 -> [w90]
        tunnel: [w89] -> w29 mode=indexing
        tunnel: w12 -> [_]
        tunnel: [errorcluster {"status"=FALSE, "code"=0, "source"=""} ("error in")] -> w11
        i -> [w91]
        n36 = Index Array(array=w90, index=w91) -> (element=w86:T17)
        n37 = Unbundle By Name(w86) -> ("Timeout"=w85:u32)
        n38 = Greater?(x=w85, y=u32 1000) -> (0:w84:bool)
        n39 = case shown="False" w84 {
          tunnel: [w92 1000] -> w87
          tunnel: w85 -> [w92 _]
          frame False {
          }
          frame True {
          }
        }
        n40 = Bundle By Name(cluster=w86, "Timeout"=w87) -> (w89:T17)
      }
      n41 = call "Unbunde/bundle interface clusters for PI Terminal.vi"("System No."="System No.", "Interface configuration"=w29, "DLL Interface\nconfiguration"=w9, "TCP/IP Configuration"=w26, "Flow control"=w24, "Termination character"=w25) -> ("Term.char"=→"Term.char":T5, "TCP/IP Config. System"=→"TCP/IP Config. System":T1, "Interface"=w33:T10, "RS232 configuration system"=→"RS232 Config. System":T18, "GPIB configuration system"=→"GPIB Configuration system":T3, "DLL for Device"=→"DLL for Device":T6, "DLL interface"=w32:T12)  [unwired: 7 out]
      "Interface" <- w33
      n42 = case shown="2" w33 {
        tunnel: w32 -> [_ _ _ w61]
        frame 0, Default {
          w54 = FALSE ("Write Attribute")
          w55 = TRUE ("Write Attribute")
          # "Rs-232"
          n43 = property on="System ind." class="DigNum (strict)"("Visible"=w55) -> ()  [unwired: 2 in, 2 out]
          n44 = property on="RS232 Config. System" class="Clust (strict)"("Visible"=w55) -> ()  [unwired: 2 in, 2 out]
          n45 = property on="GPIB Configuration system" class="Clust (strict)"("Visible"=w54) -> ()  [unwired: 2 in, 2 out]
          n46 = property on="TCP/IP Config. System" class="Clust (strict)"("Visible"=w54) -> ()  [unwired: 2 in, 2 out]
          n47 = property on="DLL for Device" class="Ring (strict)"("Visible"=w54) -> ()  [unwired: 2 in, 2 out]
        }
        frame 3 {
          w56 = FALSE ("Write Attribute")
          w57 = TRUE ("Write Attribute")
          # "TCP/IP"
          n48 = property on="System ind." class="DigNum (strict)"("Visible"=w57) -> ()  [unwired: 2 in, 2 out]
          n49 = property on="TCP/IP Config. System" class="Clust (strict)"("Visible"=w57) -> ()  [unwired: 2 in, 2 out]
          n50 = property on="GPIB Configuration system" class="Clust (strict)"("Visible"=w56) -> ()  [unwired: 2 in, 2 out]
          n51 = property on="DLL for Device" class="Ring (strict)"("Visible"=w56) -> ()  [unwired: 2 in, 2 out]
          n52 = property on="RS232 Config. System" class="Clust (strict)"("Visible"=w56) -> ()  [unwired: 2 in, 2 out]
        }
        frame 1 {
          w59 = TRUE ("Write Attribute")
          w58 = FALSE ("Write Attribute")
          # "GPIB"
          n53 = property on="GPIB Configuration system" class="Clust (strict)"("Visible"=w59) -> ()  [unwired: 2 in, 2 out]
          n54 = property on="System ind." class="DigNum (strict)"("Visible"=w59) -> ()  [unwired: 2 in, 2 out]
          n55 = property on="TCP/IP Config. System" class="Clust (strict)"("Visible"=w58) -> ()  [unwired: 2 in, 2 out]
          n56 = property on="RS232 Config. System" class="Clust (strict)"("Visible"=w58) -> ()  [unwired: 2 in, 2 out]
          n57 = property on="DLL for Device" class="Ring (strict)"("Visible"=w58) -> ()  [unwired: 2 in, 2 out]
        }
        frame 2 {
          # "DLL"
          n58 = property on="DLL for Device" class="Ring (strict)"("Visible"=TRUE ("Write Attribute")) -> ()  [unwired: 2 in, 2 out]
          n59 = case shown="7" w61 {
            frame 0, Default {
              w62 = FALSE ("Write Attribute")
              w63 = TRUE ("Write Attribute")
              # "RS-232"
              n60 = property on="RS232 Config. System" class="Clust (strict)"("Visible"=w63) -> ()  [unwired: 2 in, 2 out]
              n61 = property on="System ind." class="DigNum (strict)"("Visible"=w63) -> ()  [unwired: 2 in, 2 out]
              n62 = property on="GPIB Configuration system" class="Clust (strict)"("Visible"=w62) -> ()  [unwired: 2 in, 2 out]
              n63 = property on="TCP/IP Config. System" class="Clust (strict)"("Visible"=w62) -> ()  [unwired: 2 in, 2 out]
            }
            frame 1 {
              w65 = TRUE ("Write Attribute")
              w64 = FALSE ("Write Attribute")
              # "GPIB"
              n64 = property on="GPIB Configuration system" class="Clust (strict)"("Visible"=w65) -> ()  [unwired: 2 in, 2 out]
              n65 = property on="System ind." class="DigNum (strict)"("Visible"=w65) -> ()  [unwired: 2 in, 2 out]
              n66 = property on="RS232 Config. System" class="Clust (strict)"("Visible"=w64) -> ()  [unwired: 2 in, 2 out]
              n67 = property on="TCP/IP Config. System" class="Clust (strict)"("Visible"=w64) -> ()  [unwired: 2 in, 2 out]
            }
            frame 2 {
              w66 = FALSE ("Write Attribute")
              # "Board"
              n68 = property on="TCP/IP Config. System" class="Clust (strict)"("Visible"=w66) -> ()  [unwired: 2 in, 2 out]
              n69 = property on="GPIB Configuration system" class="Clust (strict)"("Visible"=w66) -> ()  [unwired: 2 in, 2 out]
              n70 = property on="RS232 Config. System" class="Clust (strict)"("Visible"=w66) -> ()  [unwired: 2 in, 2 out]
              n71 = property on="System ind." class="DigNum (strict)"("Visible"=w66) -> ()  [unwired: 2 in, 2 out]
            }
            frame 3 {
              w68 = FALSE ("Write Attribute")
              # "TCPIP"
              n72 = property on="TCP/IP Config. System" class="Clust (strict)"("Visible"=TRUE) -> ()  [unwired: 2 in, 2 out]
              n73 = property on="GPIB Configuration system" class="Clust (strict)"("Visible"=w68) -> ()  [unwired: 2 in, 2 out]
              n74 = property on="RS232 Config. System" class="Clust (strict)"("Visible"=w68) -> ()  [unwired: 2 in, 2 out]
              n75 = property on="System ind." class="DigNum (strict)"("Visible"=w68) -> ()  [unwired: 2 in, 2 out]
            }
            frame 7 {
              w70 = FALSE ("Write Attribute")
              # "TCPIP_DC"
              n76 = property on="TCP/IP Config. System" class="Clust (strict)"("Visible"=TRUE) -> ()  [unwired: 2 in, 2 out]
              n77 = property on="GPIB Configuration system" class="Clust (strict)"("Visible"=w70) -> ()  [unwired: 2 in, 2 out]
              n78 = property on="RS232 Config. System" class="Clust (strict)"("Visible"=w70) -> ()  [unwired: 2 in, 2 out]
              n79 = property on="System ind." class="DigNum (strict)"("Visible"=w70) -> ()  [unwired: 2 in, 2 out]
            }
            frame 4 {
              w72 = FALSE ("Write Attribute")
              # "USB"
              n80 = property on="TCP/IP Config. System" class="Clust (strict)"("Visible"=FALSE) -> ()  [unwired: 2 in, 2 out]
              n81 = property on="GPIB Configuration system" class="Clust (strict)"("Visible"=w72) -> ()  [unwired: 2 in, 2 out]
              n82 = property on="RS232 Config. System" class="Clust (strict)"("Visible"=w72) -> ()  [unwired: 2 in, 2 out]
              n83 = property on="System ind." class="DigNum (strict)"("Visible"=w72) -> ()  [unwired: 2 in, 2 out]
            }
            frame 5 {
              w73 = FALSE ("Write Attribute")
              w74 = TRUE ("Write Attribute")
              # "RS232_DC"
              n84 = property on="RS232 Config. System" class="Clust (strict)"("Visible"=w74) -> ()  [unwired: 2 in, 2 out]
              n85 = property on="System ind." class="DigNum (strict)"("Visible"=w74) -> ()  [unwired: 2 in, 2 out]
              n86 = property on="GPIB Configuration system" class="Clust (strict)"("Visible"=w73) -> ()  [unwired: 2 in, 2 out]
              n87 = property on="TCP/IP Config. System" class="Clust (strict)"("Visible"=w73) -> ()  [unwired: 2 in, 2 out]
            }
            frame 6 {
              w76 = FALSE ("Write Attribute")
              # "USB_DC"
              n88 = property on="TCP/IP Config. System" class="Clust (strict)"("Visible"=FALSE) -> ()  [unwired: 2 in, 2 out]
              n89 = property on="GPIB Configuration system" class="Clust (strict)"("Visible"=w76) -> ()  [unwired: 2 in, 2 out]
              n90 = property on="RS232 Config. System" class="Clust (strict)"("Visible"=w76) -> ()  [unwired: 2 in, 2 out]
              n91 = property on="System ind." class="DigNum (strict)"("Visible"=w76) -> ()  [unwired: 2 in, 2 out]
            }
          }
        }
      }
      n92 = call "Initialize Global1.vi"("System no."=w13, "error in"=w11) -> ("error out"=w22:errorcluster)  [unwired: 17 out]
      n93 = call "Initialize Global DaisyChain.vi"("System no."=w13, "error in"=w22) -> ("error out"=w4:errorcluster)  [unwired: 17 out]
      n94 = Initialize Array("XXX\n", w13) -> (w15:string[])
      n95 = Initialize Array(T7 {"data bits"=8, "stop bits"=enum."1 bit", "parity"=enum."no parity"} ("Bit settings and parity"), w13) -> (w17:T19)
      n96 = Initialize Array(FALSE ("Register DC"), w13) -> (w21:bool[])
      n97 = Initialize Array("ERR?", w13) -> (w19:string[])
      n98 = call "PI Open Interface.vi"("Interface clear"=w15, "Number of systems"=w13, "Interface configuration"=w29, "Strings to send"=w19, "error in"=w40, "DLL Interface\nConfiguration"=w9, "Bit settings and parity"=w17, "TCP/IP\nConfiguration"=w26, "Flow control"=w24, "Termination character"=w25, "Syntax"=w23, "Register DC"=w21) -> ("error out"=w39:errorcluster)  [unwired: 7 out]
      n99 = Unbundle By Name(w39) -> ("status"=w31:bool, "code"=w37:i32, "source"=w36:string)
      "error" <- w31
      n100 = case shown="True" w31 {
        tunnel: w37 -> [_ w81]
        tunnel: w36 -> [_ w80]
        frame False {
        }
        frame True {
          n101 = Number To Decimal String(number=w81) -> (decimal integer string=w78:string)  [unwired: 1 out]
          n102 = Concatenate Strings(w80, " , Code: " ("Substring"), w78) -> (w77:string)
          n103 = One Button Dialog(message=w77) -> (true=w82:bool)  [unwired: 1 out]
          n104 = Stop(stop? (T)=w82) -> ()
        }
      }
      "System ind." <- "System No."
      "System" <- "System No."
    }
    frame #2 {
      n105 = property on="System No." class="DigNum (strict)"("Visible"=TRUE ("Write Attribute")) -> ()  [unwired: 2 in, 2 out]
      n106 = while {
        tunnel: w101 -> [w116]
        tunnel: [w117] -> w102
        shift-left: 0 -> [w130]
        shift-right: [w129] -> w98
        shift-left: 0 -> [w126]
        shift-right: [w120] -> w99
        shift-left: "" -> [w127]
        shift-right: [w121] -> w100
        shift-left: "" -> [w138]
        shift-right: [w137] -> w97
        shift-left: 0 -> [w142]
        shift-right: [w141] -> w96
        tunnel: w110 -> [w146]
        tunnel: w111 -> [w147]
        shift-left: "*IDN?" -> [w144]
        shift-right: [w143] -> _
        tunnel: w95 -> [w114]
        tunnel: w94 -> [w113]
        stop <- w117 continue-if-true
        n107 = local read "System No."() -> (w135:i32)
        n108 = property on="Send" class="Str"("Key Focus"=TRUE ("Write Attribute")) -> ()  [unwired: 2 in, 2 out]
        n109 = case shown="False" "Send" {
          tunnel: w135 -> [w192 w240]
          tunnel: w147 -> [w191 _]
          tunnel: w146 -> [w190 _]
          tunnel: w144 -> [w197 w238]
          tunnel: [w197 w235] -> w143
          tunnel: w142 -> [w196 w226]
          tunnel: [w196 w223] -> w141
          tunnel: w138 -> [w193 w234]
          tunnel: [w193 w230] -> w137
          tunnel: [w196 w223] -> w136
          tunnel: w130 -> [w194 w229]
          tunnel: [w194 w225] -> w129
          tunnel: w116 -> [w186 _]
          tunnel: w114 -> [w185 _]
          tunnel: w113 -> [w184 _]
          frame False {
            n110 = local write "System ind."(w192) -> ()
            n111 = local write "System"(w192) -> ()
            n112 = call "Unbunde/bundle interface clusters for PI Terminal.vi"("System No."=w192, "Interface configuration"=w191, "DLL Interface\nconfiguration"=w190, "TCP/IP Configuration"=w185, "Flow control"=w186, "Termination character"=w184) -> ("Term.char"=w182:T5, "TCP/IP Config. System"=w183:T1, "Interface"=w181:T10, "RS232 configuration system"=w189:T18, "GPIB configuration system"=w188:T3, "DLL for Device"=w187:T6, "DLL interface"=w180:T12)  [unwired: 7 out]
            n113 = local write "TCP/IP Config. System"(w183) -> ()
            n114 = local write "GPIB Configuration system"(w188) -> ()
            n115 = local write "RS232 Config. System"(w189) -> ()
            n116 = local write "DLL for Device"(w187) -> ()
            n117 = local write "Term.char"(w182) -> ()
            n118 = local write "Interface"(w181) -> ()
            n119 = case shown="2" w181 {
              tunnel: w180 -> [_ _ _ w205]
              frame 0, Default {
                w198 = FALSE ("Write Attribute")
                w199 = TRUE ("Write Attribute")
                # "Rs-232"
                n120 = property on="System ind." class="DigNum (strict)"("Visible"=w199) -> ()  [unwired: 2 in, 2 out]
                n121 = property on="RS232 Config. System" class="Clust (strict)"("Visible"=w199) -> ()  [unwired: 2 in, 2 out]
                n122 = property on="GPIB Configuration system" class="Clust (strict)"("Visible"=w198) -> ()  [unwired: 2 in, 2 out]
                n123 = property on="TCP/IP Config. System" class="Clust (strict)"("Visible"=w198) -> ()  [unwired: 2 in, 2 out]
                n124 = property on="DLL for Device" class="Ring (strict)"("Visible"=w198) -> ()  [unwired: 2 in, 2 out]
              }
              frame 3 {
                w200 = FALSE ("Write Attribute")
                w201 = TRUE ("Write Attribute")
                # "TCP/IP"
                n125 = property on="System ind." class="DigNum (strict)"("Visible"=w201) -> ()  [unwired: 2 in, 2 out]
                n126 = property on="TCP/IP Config. System" class="Clust (strict)"("Visible"=w201) -> ()  [unwired: 2 in, 2 out]
                n127 = property on="GPIB Configuration system" class="Clust (strict)"("Visible"=w200) -> ()  [unwired: 2 in, 2 out]
                n128 = property on="DLL for Device" class="Ring (strict)"("Visible"=w200) -> ()  [unwired: 2 in, 2 out]
                n129 = property on="RS232 Config. System" class="Clust (strict)"("Visible"=w200) -> ()  [unwired: 2 in, 2 out]
              }
              frame 1 {
                w203 = TRUE ("Write Attribute")
                w202 = FALSE ("Write Attribute")
                # "GPIB"
                n130 = property on="GPIB Configuration system" class="Clust (strict)"("Visible"=w203) -> ()  [unwired: 2 in, 2 out]
                n131 = property on="System ind." class="DigNum (strict)"("Visible"=w203) -> ()  [unwired: 2 in, 2 out]
                n132 = property on="TCP/IP Config. System" class="Clust (strict)"("Visible"=w202) -> ()  [unwired: 2 in, 2 out]
                n133 = property on="RS232 Config. System" class="Clust (strict)"("Visible"=w202) -> ()  [unwired: 2 in, 2 out]
                n134 = property on="DLL for Device" class="Ring (strict)"("Visible"=w202) -> ()  [unwired: 2 in, 2 out]
              }
              frame 2 {
                # "DLL"
                n135 = property on="DLL for Device" class="Ring (strict)"("Visible"=TRUE ("Write Attribute")) -> ()  [unwired: 2 in, 2 out]
                n136 = case shown="7" w205 {
                  frame 0, Default {
                    w206 = FALSE ("Write Attribute")
                    w207 = TRUE ("Write Attribute")
                    # "RS-232"
                    n137 = property on="RS232 Config. System" class="Clust (strict)"("Visible"=w207) -> ()  [unwired: 2 in, 2 out]
                    n138 = property on="System ind." class="DigNum (strict)"("Visible"=w207) -> ()  [unwired: 2 in, 2 out]
                    n139 = property on="GPIB Configuration system" class="Clust (strict)"("Visible"=w206) -> ()  [unwired: 2 in, 2 out]
                    n140 = property on="TCP/IP Config. System" class="Clust (strict)"("Visible"=w206) -> ()  [unwired: 2 in, 2 out]
                  }
                  frame 1 {
                    w209 = TRUE ("Write Attribute")
                    w208 = FALSE ("Write Attribute")
                    # "GPIB"
                    n141 = property on="GPIB Configuration system" class="Clust (strict)"("Visible"=w209) -> ()  [unwired: 2 in, 2 out]
                    n142 = property on="System ind." class="DigNum (strict)"("Visible"=w209) -> ()  [unwired: 2 in, 2 out]
                    n143 = property on="RS232 Config. System" class="Clust (strict)"("Visible"=w208) -> ()  [unwired: 2 in, 2 out]
                    n144 = property on="TCP/IP Config. System" class="Clust (strict)"("Visible"=w208) -> ()  [unwired: 2 in, 2 out]
                  }
                  frame 2 {
                    w210 = FALSE ("Write Attribute")
                    # "Board"
                    n145 = property on="TCP/IP Config. System" class="Clust (strict)"("Visible"=w210) -> ()  [unwired: 2 in, 2 out]
                    n146 = property on="GPIB Configuration system" class="Clust (strict)"("Visible"=w210) -> ()  [unwired: 2 in, 2 out]
                    n147 = property on="RS232 Config. System" class="Clust (strict)"("Visible"=w210) -> ()  [unwired: 2 in, 2 out]
                    n148 = property on="System ind." class="DigNum (strict)"("Visible"=w210) -> ()  [unwired: 2 in, 2 out]
                  }
                  frame 3 {
                    w212 = FALSE ("Write Attribute")
                    # "TCPIP"
                    n149 = property on="TCP/IP Config. System" class="Clust (strict)"("Visible"=TRUE) -> ()  [unwired: 2 in, 2 out]
                    n150 = property on="GPIB Configuration system" class="Clust (strict)"("Visible"=w212) -> ()  [unwired: 2 in, 2 out]
                    n151 = property on="RS232 Config. System" class="Clust (strict)"("Visible"=w212) -> ()  [unwired: 2 in, 2 out]
                    n152 = property on="System ind." class="DigNum (strict)"("Visible"=w212) -> ()  [unwired: 2 in, 2 out]
                  }
                  frame 7 {
                    w214 = FALSE ("Write Attribute")
                    # "TCPIP_DC"
                    n153 = property on="TCP/IP Config. System" class="Clust (strict)"("Visible"=TRUE) -> ()  [unwired: 2 in, 2 out]
                    n154 = property on="GPIB Configuration system" class="Clust (strict)"("Visible"=w214) -> ()  [unwired: 2 in, 2 out]
                    n155 = property on="RS232 Config. System" class="Clust (strict)"("Visible"=w214) -> ()  [unwired: 2 in, 2 out]
                    n156 = property on="System ind." class="DigNum (strict)"("Visible"=w214) -> ()  [unwired: 2 in, 2 out]
                  }
                  frame 4 {
                    w216 = FALSE ("Write Attribute")
                    # "USB"
                    n157 = property on="TCP/IP Config. System" class="Clust (strict)"("Visible"=FALSE) -> ()  [unwired: 2 in, 2 out]
                    n158 = property on="GPIB Configuration system" class="Clust (strict)"("Visible"=w216) -> ()  [unwired: 2 in, 2 out]
                    n159 = property on="RS232 Config. System" class="Clust (strict)"("Visible"=w216) -> ()  [unwired: 2 in, 2 out]
                    n160 = property on="System ind." class="DigNum (strict)"("Visible"=w216) -> ()  [unwired: 2 in, 2 out]
                  }
                  frame 5 {
                    w217 = FALSE ("Write Attribute")
                    w218 = TRUE ("Write Attribute")
                    # "RS232_DC"
                    n161 = property on="RS232 Config. System" class="Clust (strict)"("Visible"=w218) -> ()  [unwired: 2 in, 2 out]
                    n162 = property on="System ind." class="DigNum (strict)"("Visible"=w218) -> ()  [unwired: 2 in, 2 out]
                    n163 = property on="GPIB Configuration system" class="Clust (strict)"("Visible"=w217) -> ()  [unwired: 2 in, 2 out]
                    n164 = property on="TCP/IP Config. System" class="Clust (strict)"("Visible"=w217) -> ()  [unwired: 2 in, 2 out]
                  }
                  frame 6 {
                    w220 = FALSE ("Write Attribute")
                    # "USB_DC"
                    n165 = property on="TCP/IP Config. System" class="Clust (strict)"("Visible"=FALSE) -> ()  [unwired: 2 in, 2 out]
                    n166 = property on="GPIB Configuration system" class="Clust (strict)"("Visible"=w220) -> ()  [unwired: 2 in, 2 out]
                    n167 = property on="RS232 Config. System" class="Clust (strict)"("Visible"=w220) -> ()  [unwired: 2 in, 2 out]
                    n168 = property on="System ind." class="DigNum (strict)"("Visible"=w220) -> ()  [unwired: 2 in, 2 out]
                  }
                }
              }
            }
            n169 = property on="Send" class="Str"("Key Focus"=TRUE ("Write Attribute")) -> ()  [unwired: 2 in, 2 out]
          }
          frame True {
            n170 = Add(x=w229, y=1) -> (x+y=w225:i32)
            n171 = local read "Send"() -> (w237:string)
            n172 = String Length(string=w237) -> (length=w231:i32)
            n173 = Subtract(x=w231, y=w226) -> (x-y=w236:i32)
            n174 = String Subset(string=w237, offset (0)=w226, length (rest)=w236) -> (substring=w232:string)
            n175 = call "Analyse input string for terminal.vi"("Last string sent"=w238, "String new"=w232) -> ("String out"=w235:string, "Out not equal to in?"=w233:bool, "Attach term. char.?"=w221:bool)  [unwired: 15 out]
            n176 = case shown="True" w233 {
              tunnel: w235 -> [w250 w256]
              tunnel: [w247 w254] -> w230
              tunnel: w234 -> [w253 w257]
              tunnel: w232 -> [w252 _]
              frame True {
                n177 = Concatenate Strings(w253, w252, "  (Sent: " ("Substring"), w250, ")" ("Substring"), "\n") -> (w247:string)
                n178 = local write "Send"(w247) -> ()
              }
              frame False {
                n179 = Concatenate Strings(w257, w256, "\n") -> (w254:string)
                n180 = local write "Send"(w254) -> ()
              }
            }
            n181 = stacked-sequence {
              tunnel: [w245] -> w227
              tunnel: w230 -> [w246]
              frame #0 {
                n182 = String Length(string=w246) -> (length=w245:i32)
                n183 = property on="Send" class="Str"("Text.Selection:Start"=w245, "Text.Selection:End"=w245) -> ()  [unwired: 2 in, 2 out]
              }
            }
            n184 = stacked-sequence {
              tunnel: w227 -> [w242]
              tunnel: [w242] -> w224
              tunnel: w225 -> [w241]
              frame #0 {
                n185 = property on="Send" class="Str"("Text.Scroll Position"=w241) -> ()  [unwired: 2 in, 2 out]
              }
            }
            n186 = call "PI Send String.vi"("System no."=w240, "String to send"=w235, "Attach termination char.?"=w221) -> ("error out"=w222:errorcluster)  [unwired: 1 in, 15 out]
            "error out" <- w222
            n187 = stacked-sequence {
              tunnel: w224 -> [w243]
              tunnel: [w243] -> w223
              tunnel: w222 -> [_]
              frame #0 {
                n188 = property on="Send" class="Str"("Key Focus"=TRUE ("Write Attribute")) -> ()  [unwired: 2 in, 2 out]
              }
            }
            n189 = Unbundle By Name(w222) -> ("status"=w239:bool)
            n190 = local write "error"(w239) -> ()
          }
        }
        n191 = case shown="False" "Clear" {
          tunnel: [w158 ""] -> w124
          tunnel: w127 -> [w158 _]
          tunnel: [w157 0] -> w125
          tunnel: w126 -> [w157 _]
          frame False {
          }
          frame True {
            n192 = local write "Receive"("") -> ()
          }
        }
        n193 = case shown="0, Default" "View style" {
          tunnel: [u32 0 ("Write Attribute") u32 1 ("Write Attribute") u32 3 ("Write Attribute")] -> w139
          frame 0, Default {
          }
          frame 1 {
          }
          frame 2 {
          }
        }
        n194 = stacked-sequence {
          tunnel: w136 -> [_]
          tunnel: w135 -> [w176]
          tunnel: [w175] -> w134
          tunnel: [w174] -> w132
          tunnel: w124 -> [_]
          frame #0 {
            n195 = call "PI Receive String.vi"("System no."=w176, "Strip spaces?"=FALSE) -> ("String read"=w174:string, "bytes read"=w175:u16)  [unwired: 1 in, 15 out]
          }
        }
        n196 = property on="Receive" class="Str"("Display Style"=w139) -> ()  [unwired: 2 in, 2 out]
        n197 = Greater?(x=w134, y=u16 1) -> (0:w123:bool)
        n198 = case shown="True" w123 {
          tunnel: [w163 w169] -> w122
          tunnel: w132 -> [_ w171]
          tunnel: w124 -> [w163 w172]
          tunnel: [w162 w167] -> w120
          tunnel: w125 -> [w162 w168]
          frame False {
          }
          frame True {
            n199 = Concatenate Strings(w172, w171, "\n" ("string")) -> (w169:string)
            n200 = call "How often does string contain regular expression?.vi"("Regular expression"="\\n" ("regular expression"), "String"=w171) -> ("Number"=w166:i32)  [unwired: 17 out]
            n201 = Increment(x=w166) -> (x+1=w164:i32)
            n202 = local write "Receive"(w169) -> ()
            n203 = Add(x=w164, y=w168) -> (x+y=w167:i32)
          }
        }
        n204 = case shown="True" "Show help" {
          frame False {
          }
          frame True {
            n205 = property on="Send" class="Str"("Visible"=FALSE ("Write Attribute")) -> ()  [unwired: 2 in, 2 out]
            n206 = property on="String" class="Str"("Visible"=TRUE ("Write Attribute")) -> ()  [unwired: 2 in, 2 out]
            n207 = while {
              tunnel: [w152] -> w149
              stop <- w152 continue-if-true
              n208 = Not(x="Hide help") -> (.not. x?=w152:bool)
            }
            n209 = Not(x=w149) -> (.not. x?=w148:bool)
            n210 = property on="Send" class="Str"("Visible"=w148) -> ()  [unwired: 2 in, 2 out]
            n211 = property on="String" class="Str"("Visible"=w149) -> ()  [unwired: 2 in, 2 out]
          }
        }
        n212 = case shown="False" w123 {
          tunnel: w122 -> [w154 w156]
          tunnel: [w154 w156] -> w121
          tunnel: w120 -> [_ w155]
          frame False {
          }
          frame True {
            n213 = property on="Receive" class="Str"("Text.Scroll Position"=w155) -> ()  [unwired: 2 in, 2 out]
          }
        }
        n214 = local read "Exit"() -> (w118:bool)
        n215 = Not(x=w118) -> (.not. x?=w117:bool)
        n216 = Wait Until Next ms Multiple(millisecond multiple=u32 10) -> ()  [unwired: 1 out]
      }
      n217 = property on="Send" class="Str"("Key Focus"=TRUE ("Write Attribute")) -> ()  [unwired: 2 in, 2 out]
      n218 = local write "Exit"(w102) -> ()
    }
    frame #3 {
      n219 = case shown="True" "ERR? on exit?" {
        tunnel: w265 -> [_ w297]
        tunnel: w264 -> [_ w296]
        tunnel: w263 -> [_ w295]
        tunnel: w262 -> [_ w294]
        tunnel: w261 -> [_ w293]
        tunnel: ["" w270] -> w258
        frame False {
        }
        frame True {
          n220 = local read "System No."() -> (w289:i32)
          n221 = Add(x=w295, y=1) -> (x+y=w285:i32)
          n222 = local read "Send"() -> (w280:string)
          n223 = String Length(string=w280) -> (length=w277:i32)
          n224 = Subtract(x=w277, y=w297) -> (x-y=w279:i32)
          n225 = String Subset(string=w280, offset (0)=w297, length (rest)=w279) -> (substring=w278:string)
          n226 = call "Analyse input string for terminal.vi"("Last string sent"="ERR?", "String new"=w278) -> ("String out"=w292:string)  [unwired: 17 out]
          n227 = Concatenate Strings(w296, w278, "  (Sent: " ("Substring"), w292, ")" ("Substring"), "\n") -> (w291:string)
          n228 = stacked-sequence {
            tunnel: [w303] -> w275
            tunnel: w291 -> [w304]
            frame #0 {
              n229 = String Length(string=w304) -> (length=w303:i32)
              n230 = property on="Send" class="Str"("Text.Selection:Start"=w303, "Text.Selection:End"=w303) -> ()  [unwired: 2 in, 2 out]
            }
          }
          n231 = stacked-sequence {
            tunnel: w275 -> [w300]
            tunnel: [w300] -> w274
            tunnel: w285 -> [w299]
            frame #0 {
              n232 = property on="Send" class="Str"("Text.Scroll Position"=w299) -> ()  [unwired: 2 in, 2 out]
            }
          }
          n233 = stacked-sequence {
            tunnel: w274 -> [w301]
            tunnel: [w301] -> w290
            frame #0 {
              n234 = property on="Send" class="Str"("Key Focus"=TRUE ("Write Attribute")) -> ()  [unwired: 2 in, 2 out]
            }
          }
          n235 = stacked-sequence {
            tunnel: w290 -> [_]
            tunnel: w289 -> [w319]
            tunnel: [w318] -> w288
            tunnel: [w317] -> w286
            tunnel: w294 -> [_]
            frame #0 {
              n236 = call "PI Receive String.vi"("System no."=w319) -> ("String read"=w317:string, "bytes read"=w318:u16)  [unwired: 2 in, 15 out]
            }
          }
          n237 = Greater?(x=w288, y=u16 1) -> (0:w284:bool)
          n238 = case shown="True" w284 {
            tunnel: [w309 w313] -> w283
            tunnel: w286 -> [_ w315]
            tunnel: w294 -> [w309 w316]
            tunnel: [w308 w310] -> w282
            tunnel: w293 -> [w308 w311]
            frame False {
            }
            frame True {
              n239 = Concatenate Strings(w316, w315) -> (w313:string)
              n240 = call "How often does string contain regular expression?.vi"("Regular expression"="\\n" ("regular expression"), "String"=w315) -> ("Number"=w312:i32)  [unwired: 17 out]
              n241 = local write "Receive"(w313) -> ()
              n242 = Add(x=w312, y=w311) -> (x+y=w310:i32)
            }
          }
          n243 = local write "Send"(w291) -> ()
          n244 = call "PI Send String.vi"("System no."=w289, "String to send"=w292, "Attach termination char.?"=TRUE ("Attach Linefeed?")) -> ()  [unwired: 1 in, 16 out]
          n245 = case shown="True" w284 {
            tunnel: w283 -> [w305 w307]
            tunnel: [w305 w307] -> w270
            tunnel: w282 -> [_ w306]
            frame False {
            }
            frame True {
              n246 = property on="Receive" class="Str"("Text.Scroll Position"=w306) -> ()  [unwired: 2 in, 2 out]
            }
          }
        }
      }
      n247 = for {
        N: w259 -> [_]
        tunnel: w258 -> [_]
        i -> [w268]
        n248 = Increment(x=w268) -> (x+1=w267:i32)
        n249 = call "Close connection if open.vi"("System no."=w267, "Close DaisyChain"=TRUE) -> ()  [unwired: 1 in, 17 out]
      }
    }
  }
